vi "OSQ_load_legacy.vi"(8 "error in (no error)":errorcluster, 11 "XML Elements":string) -> (0 "error out":errorcluster, 2 "SEQs":T1[](array[typedef]))   [LabVIEW 2013]
uses:
  Line.ctl
panel:
  in  "Line":T1
  in  "SEQs":cluster{"Var Array":string[][]}[](array[cluster])
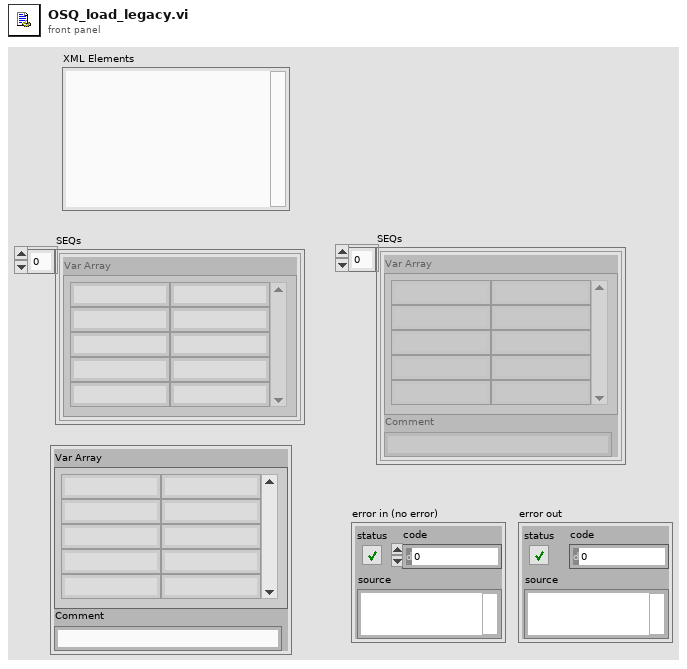
[diagram p1: front panel]
types:
  T1 = typedef "Line.ctl" = cluster{"Var Array":string[][], "Comment":string}
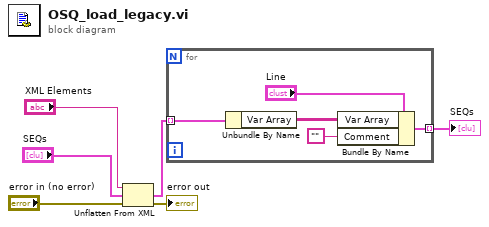
[diagram p0: block diagram]
diagram:
  n1 = Unflatten From XML(xml string="XML Elements", type="SEQs", error in (no error)="error in (no error)") -> (value=w3:cluster{"Var Array":string[][]}[], error out=→"error out":errorcluster)
  n2 = for {
    tunnel: w3 -> [w11] mode=indexing
    tunnel: [w8] -> w2 mode=indexing
    n3 = Unbundle By Name(w11) -> ("Var Array"=w9:string[][])
    n4 = Bundle By Name(cluster="Line", "Var Array"=w9, "Comment"="") -> (w8:T1)
  }
  "SEQs" <- w2
